vi "Island.vi"(8 "error in (no error)":errorcluster, 11 "SCADA in":refnum<class "SCADA.lvclass">) -> (0 "error out":errorcluster, 3 "SCADA out":refnum<class "SCADA.lvclass">)   [LabVIEW 2015, in "SCADA Core.lvlib" / "SCADA.lvclass"]
uses:
  SCADA.lvclass
  SCADA.lvclass/SCADA.ctl
  IED Actor/IED/Controls/Device Deactivate Mode Select.ctl
  IED Actor/IED Messages/Device Deactivate Msg/Device Deactivate Msg.lvclass/Device Deactivate Msg.ctl
  <vilib>/ActorFramework/Message Enqueuer/Message Enqueuer.lvclass/Message Enqueuer.ctl
  SCADA Abstract Messages/Simple Command Status Msg/Simple Command Status.ctl
  <vilib>/ActorFramework/Actor/Actor.lvclass/Actor.ctl
  <vilib>/Utility/error.llb/DialogType.ctl
  SCADA Messages/Return Island Status Msg/Return Island Status Msg.lvclass/Return Island Status Msg.ctl
  <vilib>/ActorFramework/Message Enqueuer/Enqueue.vi
  <vilib>/ActorFramework/Message Enqueuer/Init from Existing Queue.vi
  <vilib>/ActorFramework/Message Priority Queue/Priority Enqueue.vi
  IED Actor/IED Messages/Device Deactivate Msg/Device Deactivate Msg.lvclass
  <vilib>/ActorFramework/Message Enqueuer/Message Enqueuer.lvclass
  SCADA Messages/Return Island Status Msg/Return Island Status Msg.lvclass
  SCADA Abstract Messages/Simple Command Status Msg/Simple Command Status Msg.lvclass
  <vilib>/ActorFramework/Actor/Actor.lvclass
  IED Actor/IED/IED.lvclass
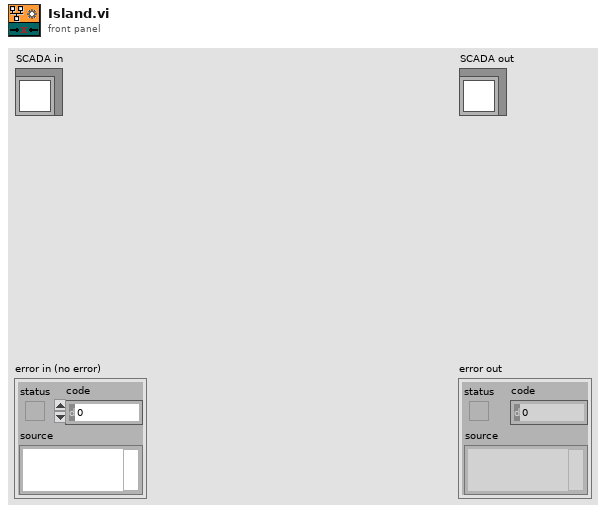
[diagram p1: front panel]
types:
  T1 = typedef "IED Actor.lvlib/IED.lvclass/Device Deactivate Mode Select.ctl" = enum16{"Deactivate", "Shutdown", "Island"}
  T2 = typedef "SCADA Core.lvlib/Simple Command Status Msg.lvclass/Simple Command Status.ctl" = enum16{"Success", "Failure"}
  T3 = typedef "SCADA Core.lvlib/SCADA.lvclass/Grid Mode.ctl" = enum16{"Off", "Grid Connected", "Islanded", "Synchronizing"}
  T4 = typedef "DialogType.ctl" = u16
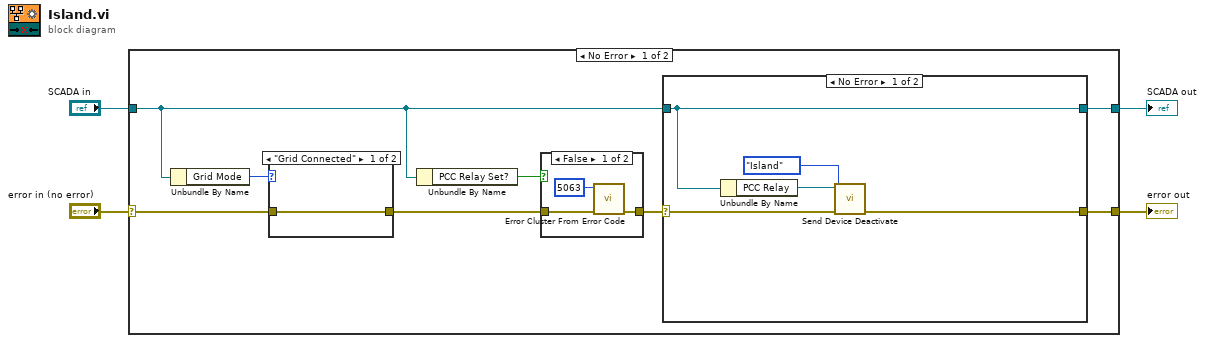
[diagram p0: block diagram]
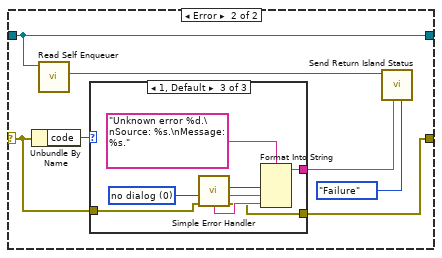
[diagram p2: hidden frame]
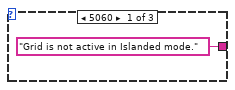
[diagram p3: hidden frame]
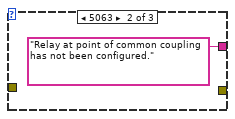
[diagram p4: hidden frame]
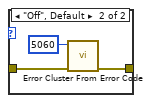
[diagram p6: hidden frame]
diagram:
  n1 = case shown="No Error" "error in (no error)" {
    selector: "error in (no error)" -> [w11 w44]
    tunnel: [w6 w44] -> w3
    tunnel: [w7 w43] -> w1
    tunnel: "SCADA in" -> [w8 w43]
    frame No Error {
      n2 = Unbundle By Name(w8) -> ("Grid Mode"=w12:T3)
      n3 = case shown="\"Grid Connected\"" w12 {
        tunnel: w11 -> [w39 w42]
        tunnel: [w39 w40] -> w5
        frame "Grid Connected" {
        }
        frame "Off", Default {
          n4 = call <vilib>:"Error Cluster From Error Code.vi"("error in (no error)"=w42, "error code (0)"=5060) -> ("error out"=w40:errorcluster)  [unwired: 7 in]
        }
      }
      n5 = Unbundle By Name(w8) -> ("PCC Relay Set?"=w10:bool)
      n6 = case shown="False" w10 {
        tunnel: w5 -> [w37 w38]
        tunnel: [w35 w38] -> w9
        frame False {
          n7 = call <vilib>:"Error Cluster From Error Code.vi"("error in (no error)"=w37, "error code (0)"=5063) -> ("error out"=w35:errorcluster)  [unwired: 7 in]
        }
        frame True {
        }
      }
      n8 = case shown="No Error" w9 {
        selector: w9 -> [w15 w23]
        tunnel: w8 -> [w17 w22]
        tunnel: [w17 w22] -> w7
        tunnel: [w14 w21] -> w6
        frame No Error {
          n9 = Unbundle By Name(w17) -> ("PCC Relay"=w16:refnum<class "Message Enqueuer.lvclass">)
          n10 = call "Send Device Deactivate.vi"("error in (no error)"=w15, "Activate Mode"=Device_Deactivate_Mode_Select."Island", "Message Enqueuer"=w16) -> ("error out"=w14:errorcluster)  [unwired: 7 in, 1 out]
        }
        frame Error {
          n11 = Unbundle By Name(w23) -> ("code"=w24:i32)
          n12 = call <vilib>:"Read Self Enqueuer.vi"("Actor"=w22) -> ("Self Enqueuer"=w20:refnum<class "Message Enqueuer.lvclass">)  [unwired: 10 in]
          n13 = case shown="1, Default" w24 {
            tunnel: w23 -> [_ _ w29]
            tunnel: ["Grid is not active in Islanded mode." "Relay at point of common coupling has not been configured." w28] -> w18
            tunnel: [_ _ w27] -> w21
            frame 5060 {
            }
            frame 5063 {
            }
            frame 1, Default {
              w30 = T4 0 items=["no dialog", "OK message", "continue or stop message", "OK message + warnings", "continue/stop + warnings"] ("type of dialog (OK msg:1)")
              n14 = call <vilib>:"Simple Error Handler.vi"("type of dialog (OK msg:1)"=w30, "error in (no error)"=w29) -> ("code out"=w32:i32, "source out"=w33:string, "error out"=w27:errorcluster, "message"=w34:string)  [unwired: 3 in, 1 out]
              n15 = Format Into String(format string="Unknown error %d.\nSource: %s.\nMessage: %s." ("Error String"), w32, w33, w34) -> (resulting string=w28:string)  [unwired: 2 in, 1 out]
            }
          }
          n16 = call "Send Return Island Status.vi"("Status"=Simple_Command_Status."Failure", "error"=w18, "Message Enqueuer"=w20) -> ()  [unwired: 7 in, 2 out]
        }
      }
    }
    frame Error {
    }
  }
  "error out" <- w3
  "SCADA out" <- w1
